vi "overlay_image_400x400.vi"(11 "Image 2":T1) -> (3 "Image":T1(plugin-control))   [LabVIEW 2015]
uses:
  <vilib>/vision/Image Controls.llb/IMAQ Image.ctl
panel:
  out "X Resolution":i32
  out "Y Resolution":i32
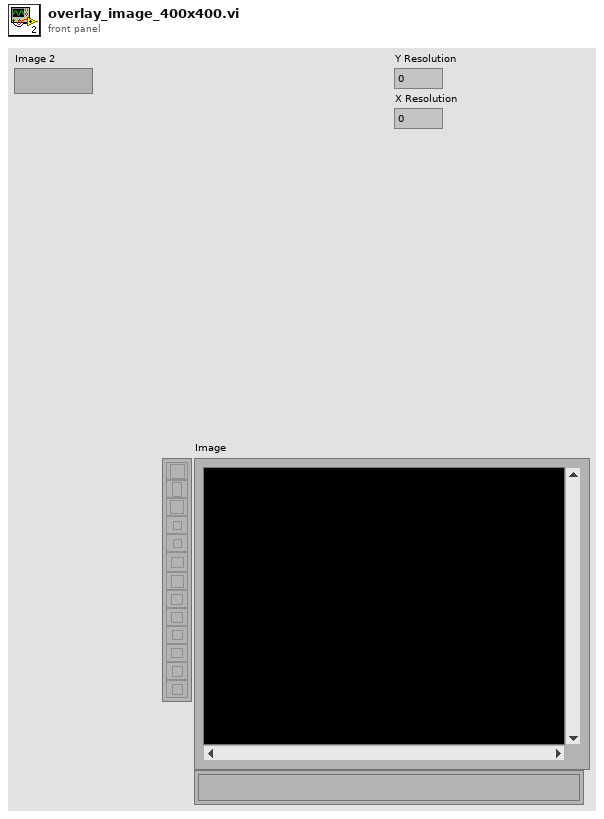
[diagram p1: front panel]
types:
  T1 = typedef "IMAQ Image.ctl" = refnum<image>
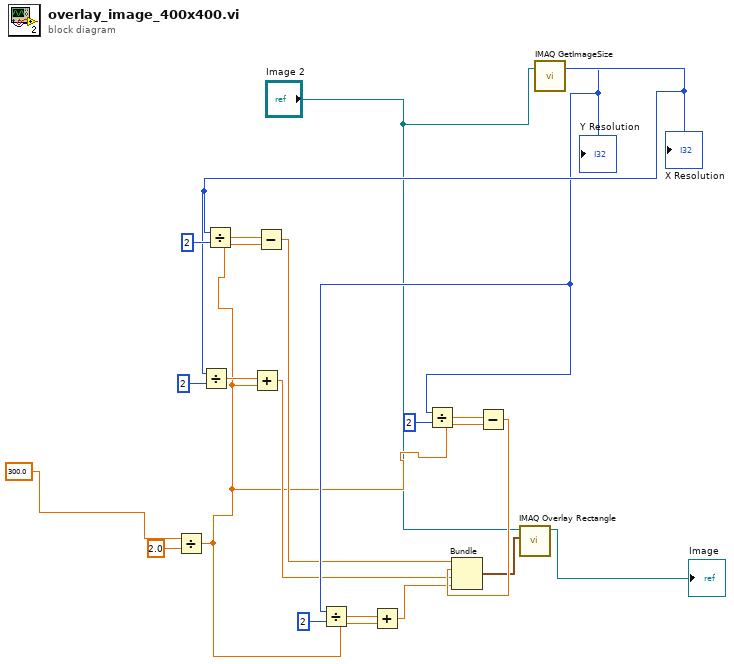
[diagram p0: block diagram]
diagram:
  n1 = Divide(x=300.0 ("Numeric"), y=2.0) -> (x/y=w3:dbl)
  n2 = call "IMAQ GetImageSize"("Image"="Image 2") -> ("Y Resolution"=w11:i32, "X Resolution"=w14:i32)  [unwired: 3 in, 1 out]
  "Y Resolution" <- w11
  "X Resolution" <- w14
  n3 = Divide(x=w14, y=2) -> (x/y=w17:dbl)
  n4 = Divide(x=w14, y=2) -> (x/y=w19:dbl)
  n5 = Add(x=w17, y=w3) -> (x+y=w7:dbl)
  n6 = Subtract(x=w19, y=w3) -> (x-y=w9:dbl)
  n7 = Divide(x=w11, y=2) -> (x/y=w12:dbl)
  n8 = Add(x=w12, y=w3) -> (x+y=w6:dbl)
  n9 = Divide(x=w11, y=2) -> (x/y=w15:dbl)
  n10 = Subtract(x=w15, y=w3) -> (x-y=w8:dbl)
  n11 = Bundle(w9, w8, w7, w6) -> (w5:cluster{dbl, dbl, dbl, dbl})  [unwired: 1 in]
  n12 = call "IMAQ Overlay Rectangle"("Rectangle"=w5, "Image"="Image 2") -> ("Image Out"=→"Image":T1)  [unwired: 8 in, 1 out]
